vi "str to uint64array.vi"(2 "String":string) -> (6 "uint64 array":u64[](array[numeric]))   [LabVIEW 2013, in "CreateOPCUAServerAuto.lvlib"]
uses:
  CreateOPCUAServerAuto.lvlib
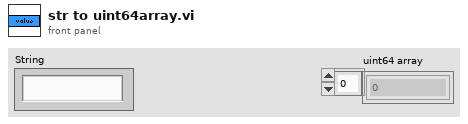
[diagram p1: front panel]
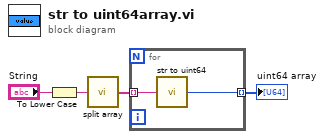
[diagram p0: block diagram]
diagram:
  n1 = To Lower Case(string="String") -> (all lower case string=w3:string)
  n2 = call "split array.vi"("string"=w3) -> ("split arr"=w2:string[])  [unwired: 8 in]
  n3 = for {
    tunnel: w2 -> [w6] mode=indexing
    tunnel: [w5] -> w1 mode=indexing
    n4 = call "str to uint64.vi"("String"=w6) -> ("uint64"=w5:u64)  [unwired: 6 in]
  }
  "uint64 array" <- w1
